vi "FindCtrl.vi"(1 "Name":string, 2 "VI":refnum<vi>, 3 "Ctrls":cluster{"Name":string, "Ctrl":refnum<vi>}[](array[cluster])) -> (0 "Ctrl":refnum<vi>)   [LabVIEW 2014]
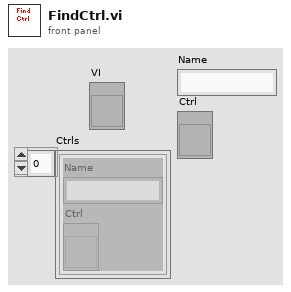
[diagram p1: front panel]
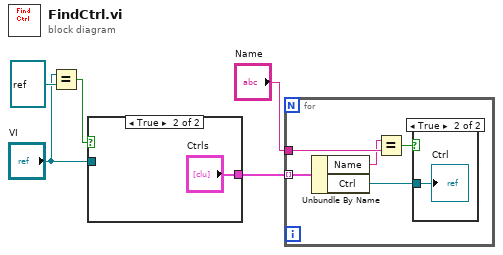
[diagram p0: block diagram]
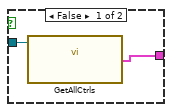
[diagram p2: hidden frame]
diagram:
  n1 = Equal?(x="VI", y=refnum<vi> refnum ("vi reference")) -> (x = y?=w3:bool)
  n2 = case shown="True" w3 {
    tunnel: "VI" -> [w7 _]
    tunnel: [w6 "Ctrls"] -> w1
    frame False {
      n3 = call "GetAllCtrls.vi"("VI"=w7) -> ("Ctrls"=w6:cluster{"Name":string, "Ctrl":refnum<vi>}[])  [unwired: 1 in]
    }
    frame True {
    }
  }
  n4 = for {
    tunnel: w1 -> [w11] mode=indexing
    tunnel: "Name" -> [w13]
    n5 = Unbundle By Name(w11) -> ("Name"=w10:string, "Ctrl"=w9:refnum<vi>)
    n6 = Equal?(x=w10, y=w13) -> (x = y?=w12:bool)
    n7 = case shown="True" w12 {
      tunnel: w9 -> [_ w14]
      frame False {
      }
      frame True {
        "Ctrl" <- w14
      }
    }
  }
